vi "special_modification.vi"(8 "error in":errorcluster, 11 "Instrument Command In":string) -> (0 "error out":errorcluster, 3 "Instrument Command Out":string)   [LabVIEW 2018]
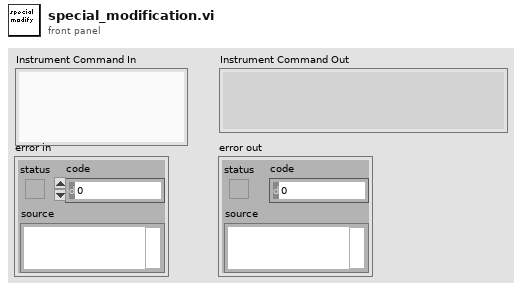
[diagram p1: front panel]
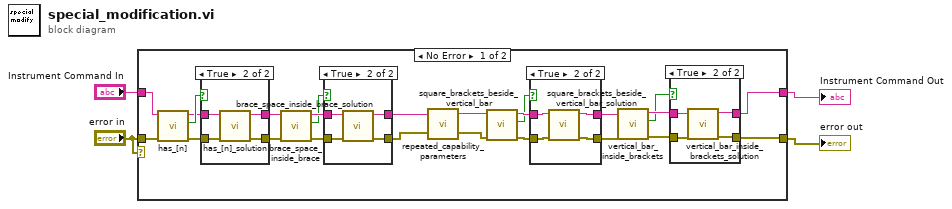
[diagram p0: block diagram]
diagram:
  n1 = case shown="No Error" "error in" {
    tunnel: [w7 w54] -> w4
    tunnel: "error in" -> [w17 w54]
    tunnel: "Instrument Command In" -> [w16 w53]
    tunnel: [w8 w53] -> w1
    frame No Error {
      n2 = call "has_[n].vi"("error in (no error)"=w17, "Instrument Command In"=w16) -> ("error out"=w20:errorcluster, "Boolean"=w19:bool, "Instrument Command Out"=w18:string)  [unwired: 7 out]
      n3 = case shown="True" w19 {
        tunnel: w18 -> [w48 w52]
        tunnel: w20 -> [w47 w51]
        tunnel: [w48 w50] -> w21
        tunnel: [w47 w49] -> w22
        frame False {
        }
        frame True {
          n4 = call "has_[n]_solution.vi"("error in (no error)"=w51, "Instrument Command In"=w52) -> ("error out"=w49:errorcluster, "Instrument Command In"=w50:string)  [unwired: 8 out]
        }
      }
      n5 = call "brace_space_inside_brace.vi"("error in (no error)"=w22, "Instrument Command In"=w21) -> ("error out"=w25:errorcluster, "Boolean"=w23:bool, "Instrument Command Out"=w24:string)  [unwired: 7 out]
      n6 = case shown="True" w23 {
        tunnel: w24 -> [w42 w46]
        tunnel: w25 -> [w41 w45]
        tunnel: [w41 w44] -> w9
        tunnel: [w42 w43] -> w10
        frame False {
        }
        frame True {
          n7 = call "brace_space_inside_brace_solution.vi"("error in (no error)"=w45, "Instrument Command In"=w46) -> ("error out"=w44:errorcluster, "Instrument Command Out"=w43:string)  [unwired: 8 out]
        }
      }
      n8 = call "repeated_capability_parameters.vi"("error in"=w9, "Instrument Command In"=w10) -> ("error out"=w5:errorcluster, "Instrument Command Out"=w6:string)
      n9 = call "square_brackets_beside_vertical_bar.vi"("error in (no error)"=w5, "Instrument Command In"=w6) -> ("error out"=w28:errorcluster, "Boolean"=w26:bool, "Instrument Command Out"=w27:string)  [unwired: 7 out]
      n10 = case shown="True" w26 {
        tunnel: w27 -> [w36 w40]
        tunnel: w28 -> [w35 w39]
        tunnel: [w35 w38] -> w14
        tunnel: [w36 w37] -> w15
        frame False {
        }
        frame True {
          n11 = call "square_brackets_beside_vertical_bar_solution.vi"("error in (no error)"=w39, "Instrument Command In"=w40) -> ("error out"=w38:errorcluster, "Instrument Command Out"=w37:string)  [unwired: 8 out]
        }
      }
      n12 = call "vertical_bar_inside_brackets.vi"("error in (no error)"=w14, "Instrument Command In"=w15) -> ("error out"=w12:errorcluster, "Boolean"=w11:bool, "Instrument Command Out"=w13:string)  [unwired: 7 out]
      n13 = case shown="True" w11 {
        tunnel: w13 -> [w30 w34]
        tunnel: w12 -> [w29 w33]
        tunnel: [w29 w32] -> w7
        tunnel: [w30 w31] -> w8
        frame False {
        }
        frame True {
          n14 = call "vertical_bar_inside_brackets_solution.vi"("error in (no error)"=w33, "Instrument Command In"=w34) -> ("error out"=w32:errorcluster, "Instrument Command Out"=w31:string)  [unwired: 8 out]
        }
      }
    }
    frame Error {
    }
  }
  "Instrument Command Out" <- w1
  "error out" <- w4
